vi "FTW-Endpoint-Listen.vi"(0 "FTW Endpoint":refnum<class "FTW-Endpoint.lvclass">, 11 "error in":errorcluster) -> (4 "FTW Endpoint out":refnum<class "FTW-Endpoint.lvclass">, 6 "New Connection":refnum<class "FTW-Endpoint.lvclass">, 15 "error out":errorcluster)   [LabVIEW 2013, in "FTW-Endpoint.lvclass"]
uses:
  FTW-Endpoint.lvclass
  FTW-Endpoint.lvclass/FTW-Endpoint.ctl
panel:
  # "Inputs"
  # "Outputs"
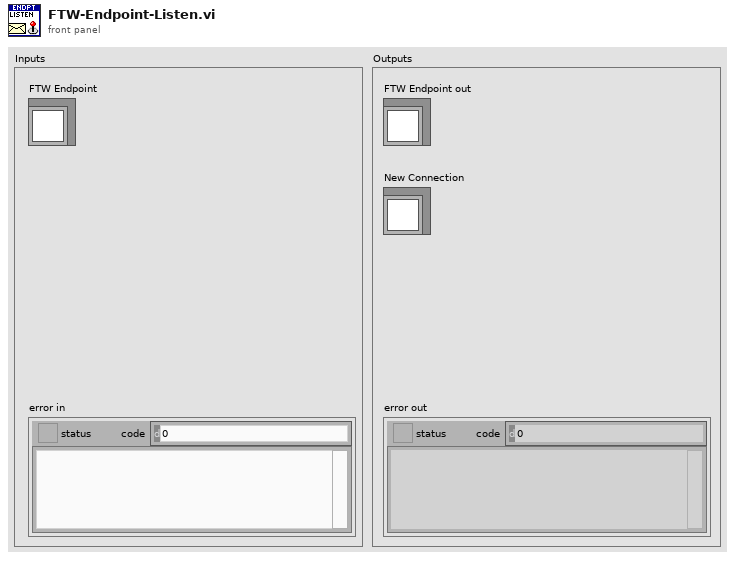
[diagram p1: front panel]
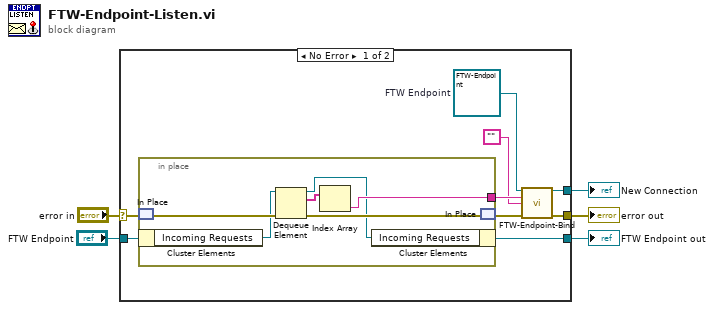
[diagram p0: block diagram]
diagram:
  n1 = case shown="No Error" "error in" {
    selector: "error in" -> [w10 w21]
    tunnel: "FTW Endpoint" -> [w9 w22]
    tunnel: [w8 w22] -> w3
    tunnel: [w7 _] -> w2
    tunnel: [w6 w21] -> w1
    frame No Error {
      w12 = refnum<class "FTW-Endpoint.lvclass"> refnum  # FTW Endpoint
      n2 = in-place {
        in-place-border: [w17] -> w13
        n3 = in-place-match #1(w10) -> (w20:errorcluster)
        n4 = in-place-cluster #2(w9) -> ("Incoming Requests"=w16:refnum<queue>)
        n5 = Dequeue Element(queue=w16, error in (no error)=w20) -> (queue out=w15:refnum<queue>, element=w18:string[], error out=w19:errorcluster)  [unwired: 1 in, 1 out]
        n6 = Index Array(array=w18) -> (element=w17:string)  [unwired: 1 in]
        n7 = in-place-cluster #2("Incoming Requests"=w15) -> (w8:refnum<class "FTW-Endpoint.lvclass">)
        n8 = in-place-match #1(w19) -> (w14:errorcluster)
      }
      n9 = call-dynamic "FTW-Endpoint-Bind.vi"("FTW Endpoint"=w12, "Endpoint Address"=w13, "Requested Identity"="", "error in"=w14) -> ("FTW Endpoint out"=w7:refnum<class "FTW-Endpoint.lvclass">, "error out"=w6:errorcluster)  [unwired: 8 in, 2 out]
    }
    frame Error {
    }
  }
  "error out" <- w1
  "FTW Endpoint out" <- w3
  "New Connection" <- w2
